vi "AIDI-Synchronize Tasks.vi"(0 "Tasks In":T1[](array[typedef]), 7 "external trig":bool, 9 "Sync task in":refnum<k21>, 11 "error in (no error)":errorcluster) -> (4 "Tasks Out":T1[](array[typedef]), 10 "Sync task out":refnum<k21>, 15 "error out":errorcluster)   [LabVIEW 2020]
uses:
  Typedefs/AIDI-Task Specification.ctl
  <vilib>/DAQmx/configure/trigger.llb/DAQmx Start Trigger (Digital Edge).vi
  <resource>/objmgr/daqmx.rc
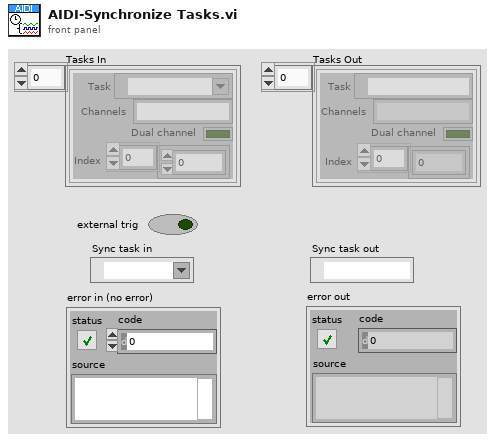
[diagram p1: front panel]
types:
  T1 = typedef "AIDI-Task Specification.ctl" = cluster{"Task":refnum<k21>, "Channels":string, "Dual channel":bool, "Index":i32[]}
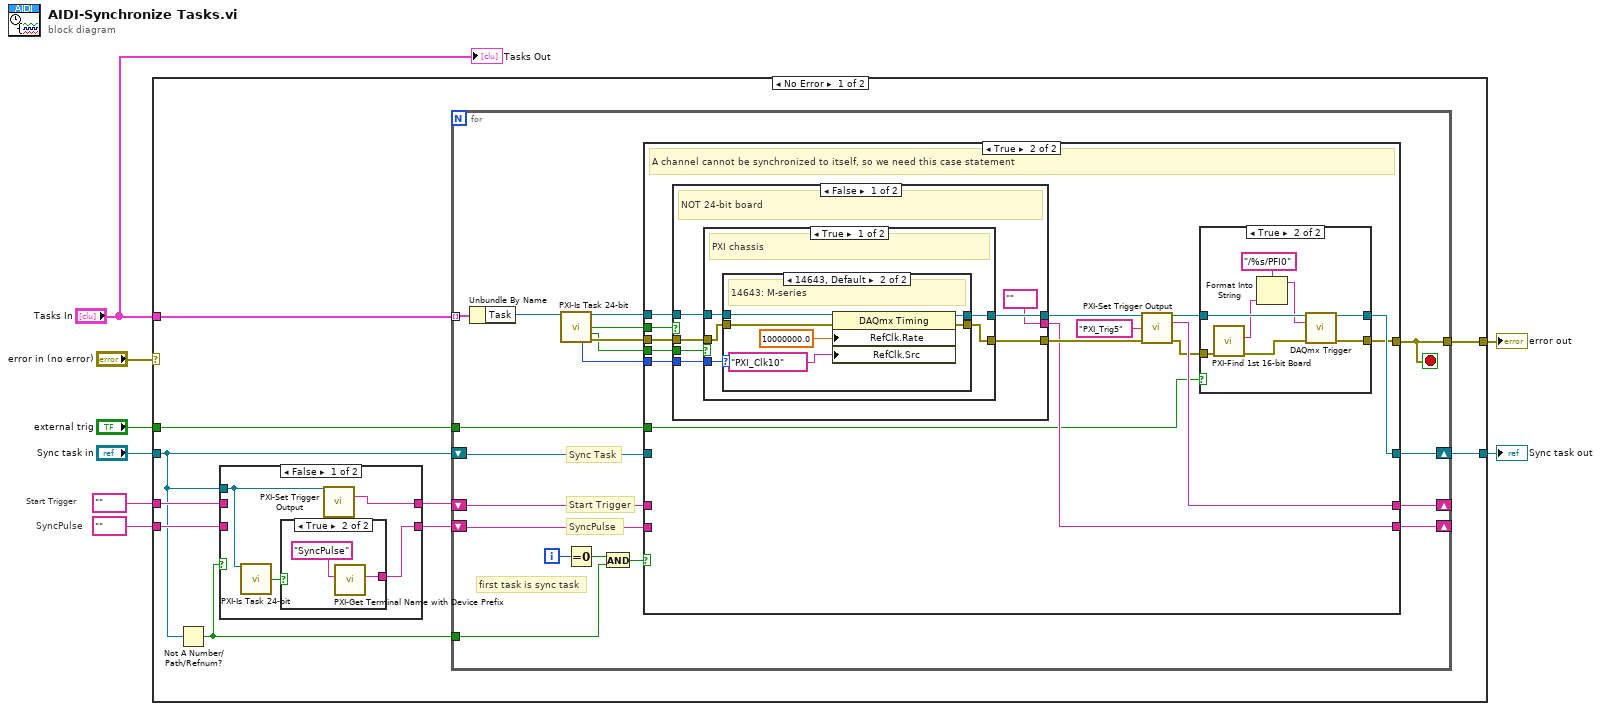
[diagram p0: block diagram]
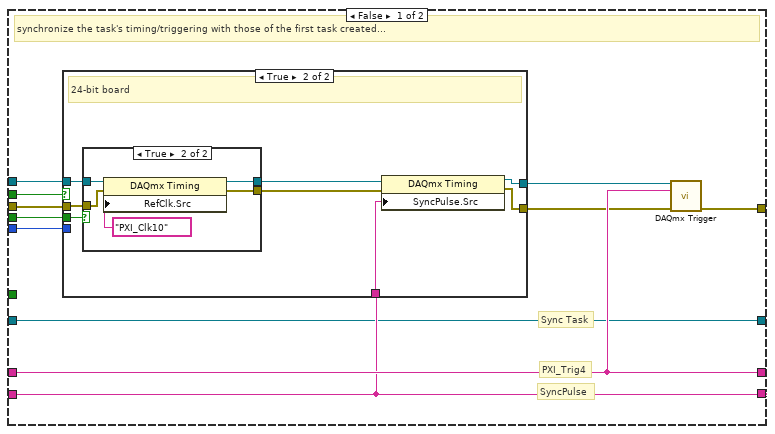
[diagram p4: hidden frame]
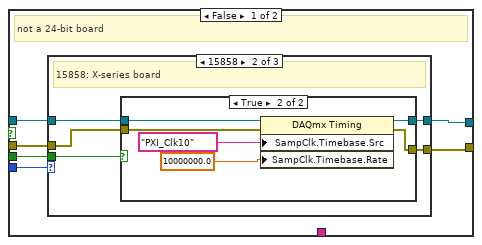
[diagram p5: hidden frame]
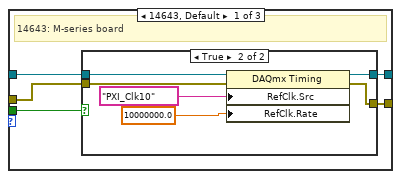
[diagram p6: hidden frame]
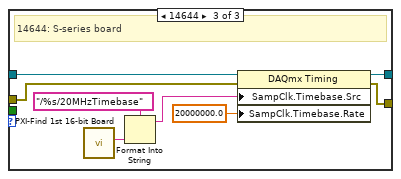
[diagram p9: hidden frame]
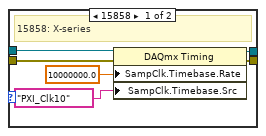
[diagram p12: hidden frame]
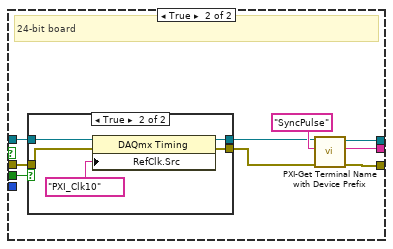
[diagram p14: hidden frame]
diagram:
  # "SyncPulse"
  # "Start Trigger"
  n1 = case shown="No Error" "error in (no error)" {
    selector: "error in (no error)" -> [_ w179]
    tunnel: "Sync task in" -> [w9 _]
    tunnel: tag "" ("source") -> [w14 _]
    tunnel: tag "" ("Terminal Name with Device Prefix") -> [w13 _]
    tunnel: "Tasks In" -> [w18 _]
    tunnel: [w17 w179] -> w3
    tunnel: [w16 _] -> w2
    tunnel: "external trig" -> [w15 _]
    frame No Error {
      n2 = Not A Number/Path/Refnum?(number/path/refnum=w9) -> (NaN/Path/Refnum?=w10:bool)
      n3 = case shown="False" w10 {
        tunnel: w14 -> [_ w26]
        tunnel: w13 -> [_ w25]
        tunnel: [w21 w26] -> w12
        tunnel: [w22 w25] -> w11
        tunnel: w9 -> [w20 _]
        frame False {
          n4 = call "PXI-Is Task 24-bit.vi"("task"=w20) -> ("is 24bit?"=w19:bool)  [unwired: 9 in, 5 out]
          n5 = case shown="True" w19 {
            tunnel: [_ w24] -> w22
            frame False {
            }
            frame True {
              n6 = call "PXI-Get Terminal Name with Device Prefix.vi"("Local Terminal Name"="SyncPulse") -> ("Terminal Name with Device Prefix"=w24:string)  [unwired: 8 in, 2 out]
            }
          }
          n7 = call "PXI-Set Trigger Output.vi"("Task in"=w20) -> ("Trigger Terminal"=w21:string)  [unwired: 12 in, 2 out]
        }
        frame True {
        }
      }
      n8 = for {
        shift-right: [w45] -> w16
        shift-left: w9 -> [w32]
        shift-right: [w43] -> _
        shift-left: w12 -> [w31]
        shift-right: [w42] -> _
        shift-left: w11 -> [w30]
        tunnel: [w37] -> w17
        tunnel: w18 -> [w34] mode=indexing
        tunnel: w15 -> [w29]
        tunnel: w10 -> [w27]
        i -> [w44]
        stop <- w37 stop-if-true
        # "SyncPulse"
        # "Start Trigger"
        # "Sync Task"
        # "first task is sync task"
        n9 = Unbundle By Name(w34) -> ("Task"=w33:refnum<k21>)
        n10 = call "PXI-Is Task 24-bit.vi"("task"=w33) -> ("task out"=w39:refnum<k21>, "is 24bit?"=w36:bool, "PXI?"=w35:bool, "Product Category"=w38:i32, "error out"=w40:errorcluster)  [unwired: 9 in, 1 out]
        n11 = Equal To 0?(x=w44) -> (x = 0?=w41:bool)
        n12 = And(x=w41, y=w27) -> (x .and. y?=w28:bool)
        n13 = case shown="True" w28 {
          tunnel: w40 -> [w54 w121]
          tunnel: [w56 w114] -> w37
          tunnel: [w48 w115] -> w45
          tunnel: w32 -> [w48 _]
          tunnel: [w55 w123] -> w43
          tunnel: w31 -> [w55 _]
          tunnel: [w53 w124] -> w42
          tunnel: w30 -> [w53 _]
          tunnel: w39 -> [w49 w122]
          tunnel: w36 -> [w50 w120]
          tunnel: w38 -> [w47 w119]
          tunnel: w35 -> [w46 w118]
          tunnel: w29 -> [_ w113]
          frame False {
            # "SyncPulse"
            # "PXI_Trig4"
            # "Sync Task"
            # "synchronize the task's timing/triggering with those of the first task created..."
            n14 = case shown="True" w50 {
              tunnel: [w60 w104] -> w52
              tunnel: [w61 w103] -> w51
              tunnel: w54 -> [w58 w102]
              tunnel: w53 -> [_ w101]
              tunnel: w49 -> [w59 w98]
              tunnel: w47 -> [w62 _]
              tunnel: w46 -> [w57 w97]
              frame False {
                # "not a 24-bit board"
                n15 = case shown="15858" w62 {
                  tunnel: [w67 w80 w96] -> w60
                  tunnel: [w66 w79 w95] -> w61
                  tunnel: w59 -> [w65 w78 w93]
                  tunnel: w58 -> [w64 w77 w92]
                  tunnel: w57 -> [w63 w76 _]
                  frame 14643, Default {
                    # "14643: M-series board"
                    n16 = case shown="True" w63 {
                      tunnel: [w69 w75] -> w67
                      tunnel: [w68 w74] -> w66
                      tunnel: w65 -> [w69 w71]
                      tunnel: w64 -> [w68 w70]
                      frame False {
                      }
                      frame True {
                        n17 = property class="DAQmx Timing"(reference=w71, error in=w70, "RefClk.Src"=tag "PXI_Clk10", "RefClk.Rate"=10000000.0) -> (reference out=w75:refnum<k21>, error out=w74:errorcluster)
                      }
                    }
                  }
                  frame 15858 {
                    # "15858: X-series board"
                    n18 = case shown="True" w76 {
                      tunnel: [w82 w88] -> w80
                      tunnel: [w81 w87] -> w79
                      tunnel: w78 -> [w82 w84]
                      tunnel: w77 -> [w81 w83]
                      frame False {
                      }
                      frame True {
                        n19 = property class="DAQmx Timing"(reference=w84, error in=w83, "SampClk.Timebase.Src"=tag "PXI_Clk10" ("RefClk.Src"), "SampClk.Timebase.Rate"=10000000.0) -> (reference out=w88:refnum<k21>, error out=w87:errorcluster)
                      }
                    }
                  }
                  frame 14644 {
                    # "14644: S-series board"
                    n20 = call "PXI-Find 1st 16-bit Board.vi"() -> ("DAQmx Device Name"=w89:tag)  [unwired: 9 in, 2 out]
                    n21 = Format Into String(format string="/%s/20MHzTimebase", w89) -> (resulting string=w90:string)  [unwired: 2 in, 1 out]
                    n22 = property class="DAQmx Timing"(reference=w93, error in=w92, "SampClk.Timebase.Src"=w90, "SampClk.Timebase.Rate"=20000000.0) -> (reference out=w96:refnum<k21>, error out=w95:errorcluster)
                  }
                }
              }
              frame True {
                # "24-bit board"
                n23 = case shown="True" w97 {
                  tunnel: w102 -> [w105 w111]
                  tunnel: [w105 w110] -> w100
                  tunnel: [w106 w109] -> w99
                  tunnel: w98 -> [w106 w108]
                  frame False {
                  }
                  frame True {
                    n24 = property class="DAQmx Timing"(reference=w108, error in=w111, "RefClk.Src"=tag "PXI_Clk10") -> (reference out=w109:refnum<k21>, error out=w110:errorcluster)
                  }
                }
                n25 = property class="DAQmx Timing"(reference=w99, error in=w100, "SyncPulse.Src"=w101) -> (reference out=w104:refnum<k21>, error out=w103:errorcluster)
              }
            }
            n26 = call-poly <vilib>:"DAQmx Trigger.vi"("task/channels in"=w52, "source"=w55, "error in"=w51) -> ("error out"=w56:errorcluster)  [unwired: 11 in, 1 out]
          }
          frame True {
            # "A channel cannot be synchronized to itself, so we need this case statement"
            n27 = case shown="False" w120 {
              tunnel: [w142 w171] -> w125
              tunnel: w122 -> [w143 w165]
              tunnel: [w141 w170] -> w126
              tunnel: w121 -> [w140 w164]
              tunnel: [tag "" ("Terminal Name with Device Prefix") w169] -> w124
              tunnel: w119 -> [w137 _]
              tunnel: w118 -> [w138 w163]
              frame False {
                # "NOT 24-bit board"
                n28 = case shown="True" w138 {
                  tunnel: w143 -> [w148 w162]
                  tunnel: [w147 w162] -> w142
                  tunnel: [w146 w161] -> w141
                  tunnel: w140 -> [w145 w161]
                  tunnel: w137 -> [w144 _]
                  frame True {
                    # "PXI chassis"
                    n29 = case shown="14643, Default" w144 {
                      tunnel: w148 -> [w154 w160]
                      tunnel: [w153 w159] -> w147
                      tunnel: [w152 w158] -> w146
                      tunnel: w145 -> [w151 w157]
                      frame 15858 {
                        # "15858: X-series"
                        n30 = property class="DAQmx Timing"(reference=w154, error in=w151, "SampClk.Timebase.Rate"=10000000.0, "SampClk.Timebase.Src"=tag "PXI_Clk10" ("RefClk.Src")) -> (reference out=w153:refnum<k21>, error out=w152:errorcluster)
                      }
                      frame 14643, Default {
                        # "14643: M-series"
                        n31 = property class="DAQmx Timing"(reference=w160, error in=w157, "RefClk.Rate"=10000000.0, "RefClk.Src"=tag "PXI_Clk10") -> (reference out=w159:refnum<k21>, error out=w158:errorcluster)
                      }
                    }
                  }
                  frame False {
                    # "NOT PXI chassis"
                  }
                }
              }
              frame True {
                # "24-bit board"
                n32 = case shown="True" w163 {
                  tunnel: [w173 w178] -> w167
                  tunnel: [w172 w177] -> w166
                  tunnel: w165 -> [w173 w176]
                  tunnel: w164 -> [w172 w175]
                  frame False {
                  }
                  frame True {
                    n33 = property class="DAQmx Timing"(reference=w176, error in=w175, "RefClk.Src"=tag "PXI_Clk10") -> (reference out=w178:refnum<k21>, error out=w177:errorcluster)
                  }
                }
                n34 = call "PXI-Get Terminal Name with Device Prefix.vi"("error in (no error)"=w166, "Local Terminal Name"="SyncPulse", "task/channels in"=w167) -> ("error out"=w170:errorcluster, "Terminal Name with Device Prefix"=w169:string, "task out"=w171:refnum<k21>)  [unwired: 6 in]
              }
            }
            n35 = call "PXI-Set Trigger Output.vi"("Task in"=w125, "Local Terminal Name"="PXI_Trig5", "error in (no error)"=w126) -> ("Task out"=w116:refnum<k21>, "Trigger Terminal"=w123:string, "error out"=w117:errorcluster)  [unwired: 10 in]
            n36 = case shown="True" w113 {
              tunnel: [w127 w136] -> w114
              tunnel: w116 -> [w128 w135]
              tunnel: w117 -> [w127 w133]
              tunnel: [w128 w134] -> w115
              frame False {
              }
              frame True {
                n37 = call "PXI-Find 1st 16-bit Board.vi"("error in (no error)"=w133) -> ("error out"=w132:errorcluster, "DAQmx Device Name"=w131:tag)  [unwired: 8 in, 1 out]
                n38 = Format Into String(format string="/%s/PFI0", w131) -> (resulting string=w129:string)  [unwired: 2 in, 1 out]
                n39 = call-poly <vilib>:"DAQmx Trigger.vi"("task/channels in"=w135, "source"=w129, "error in"=w132) -> ("task out"=w134:refnum<k21>, "error out"=w136:errorcluster)  [unwired: 11 in]
              }
            }
          }
        }
      }
    }
    frame Error {
    }
  }
  "error out" <- w3
  "Sync task out" <- w2
  "Tasks Out" <- "Tasks In"
